vi "Helium Fridge Cool-DownCaitlyn.vi"() -> ()   [LabVIEW 2014]
uses:
  <vilib>/Analysis/8numeric.llb/1D Numeric Integration.vi
  <vilib>/express/express shared/transition.llb/Dynamic To Waveform Array.vi
  <vilib>/express/express signal manip/GetorSetDDTAttributes/Set DDT Attributes/SetT0.vi
  <vilib>/express/express shared/transition.llb/Waveform Array To Dynamic.vi
  <vilib>/express/express signal manip/GetorSetDDTAttributes/Set DDT Attributes/Set DDT Properties.xnode
  <vilib>/Analysis/NI_AALPro.lvlib
panel:
  out "Array - Numeric":dbl[](array[numeric])
  out "Index":dbl
  out "Array Size":dbl
  in  "Boolean":bool
  in  "Wing Fit Subtract":bool=TRUE
  in  "Wing Fit":bool=TRUE
  out "Fit Right X":dbl[](array[numeric])
  out "Fit Left X":dbl[](array[numeric])
  out "Modulator (Y)":dbl[](array[numeric])
  out "Input Triangle (X)":dbl[](array[numeric])
  out "Fit Right Y":dbl[](array[numeric])
  out "Fit Left Y":dbl[](array[numeric])
  out "Fit Right":dbl[](array[numeric])
  out "Fit Left":dbl[](array[numeric])
  in  "Numeric Control":dbl=0.01
  out "NMR.T":dbl
  out "Temp  2":bool
  out "Q Meter Temp":dynamicdata(graph)
  in  "stop 2":bool
  in  "Right wing":dbl
  in  "Left wing":dbl
  in  "Submit":bool
  out "Is Flashing":bool
  in  "Error Beat":bool
  in  "Clear":bool
  in  "Comment":string
  out "Heartbeat":bool
  out "Most Recent Error":string
  out "Baseline Subtracted Integral vs. Time":dbl(graph)
  out "Time of Last Baseline":string
  out "Baseline":dbl[](array[numeric])
  in  "Baseline Subtract":bool
  in  "Get Baseline":bool
  out "Recording":bool
  out "Time of Last Recording":string
  in  "Record \nNMR Sweeps":bool
  in  "Depth/Div\n(kHz)":dbl=10.0
  in  "Central Freq. \n(MHz)":dbl=13.0
  in  "stop (F)":bool caption="Triangle Wave"
  in  "Triangle Wave\nRate (Hz)":dbl=0.3
  out "Time Elapsed \nDuring Sweeps (s)":dbl
  out "Lab Time":string
  out "Most Recent Error (NMR)":string
  out "Last Sweep Start Time":string
  out "Most Recent Error (Temp)":string
  out "Last Measurement Taken":string
  out "VI Start Time":string
  in  "Time Between\nTemp Ponts (s)":dbl=30.0
  out "Temp":bool
  out "NMR":bool
  in  "stop":bool
  out "Input Triangle Wave":dynamicdata(graph)
  out "Modulator":dynamicdata(graph)
  out "NMR":cluster{"Y":dbl[], "Y":dbl[]}[](graph)
  in  "# of Sweeps":dbl=1.0
  out "Resistance Strip Chart":dynamicdata(graph)
  out "Temperature Strip Chart":dynamicdata(graph)
  in  "Heartbeat":bool
  in  "Temp Strip Chart":bool
  out "Errors":bool
  in  "Silence Flashing":bool
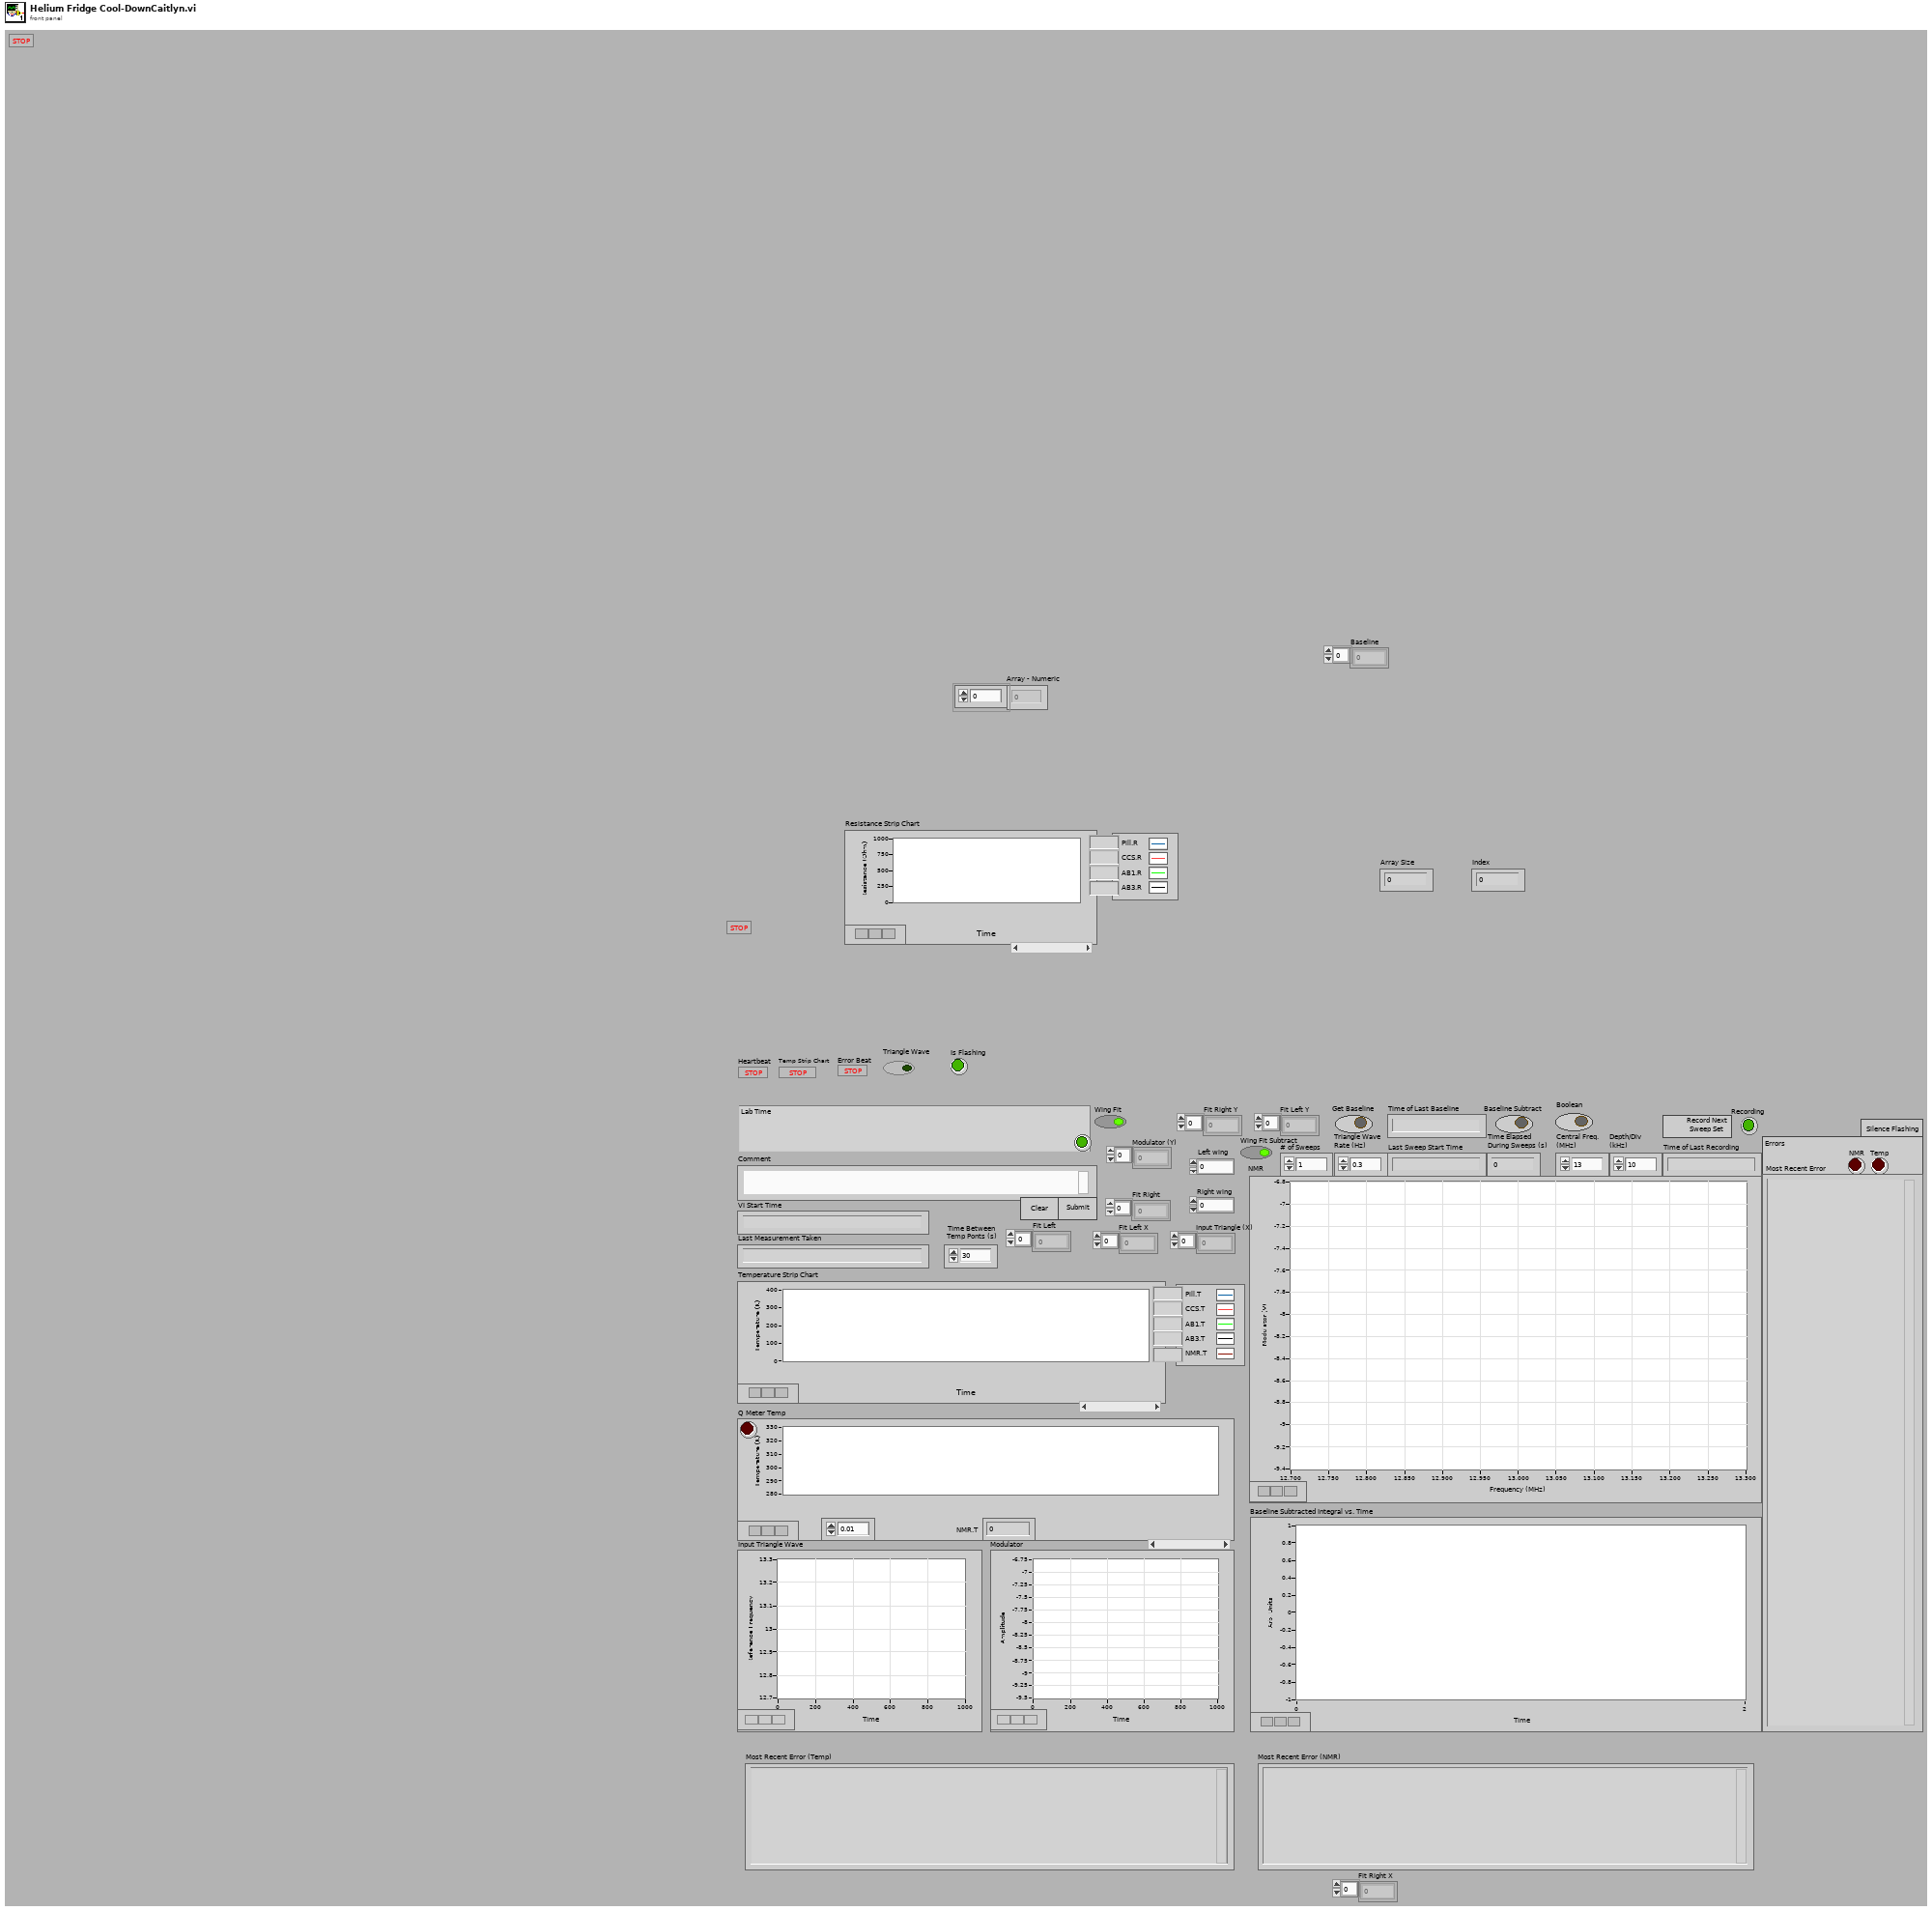
[diagram p1: front panel]
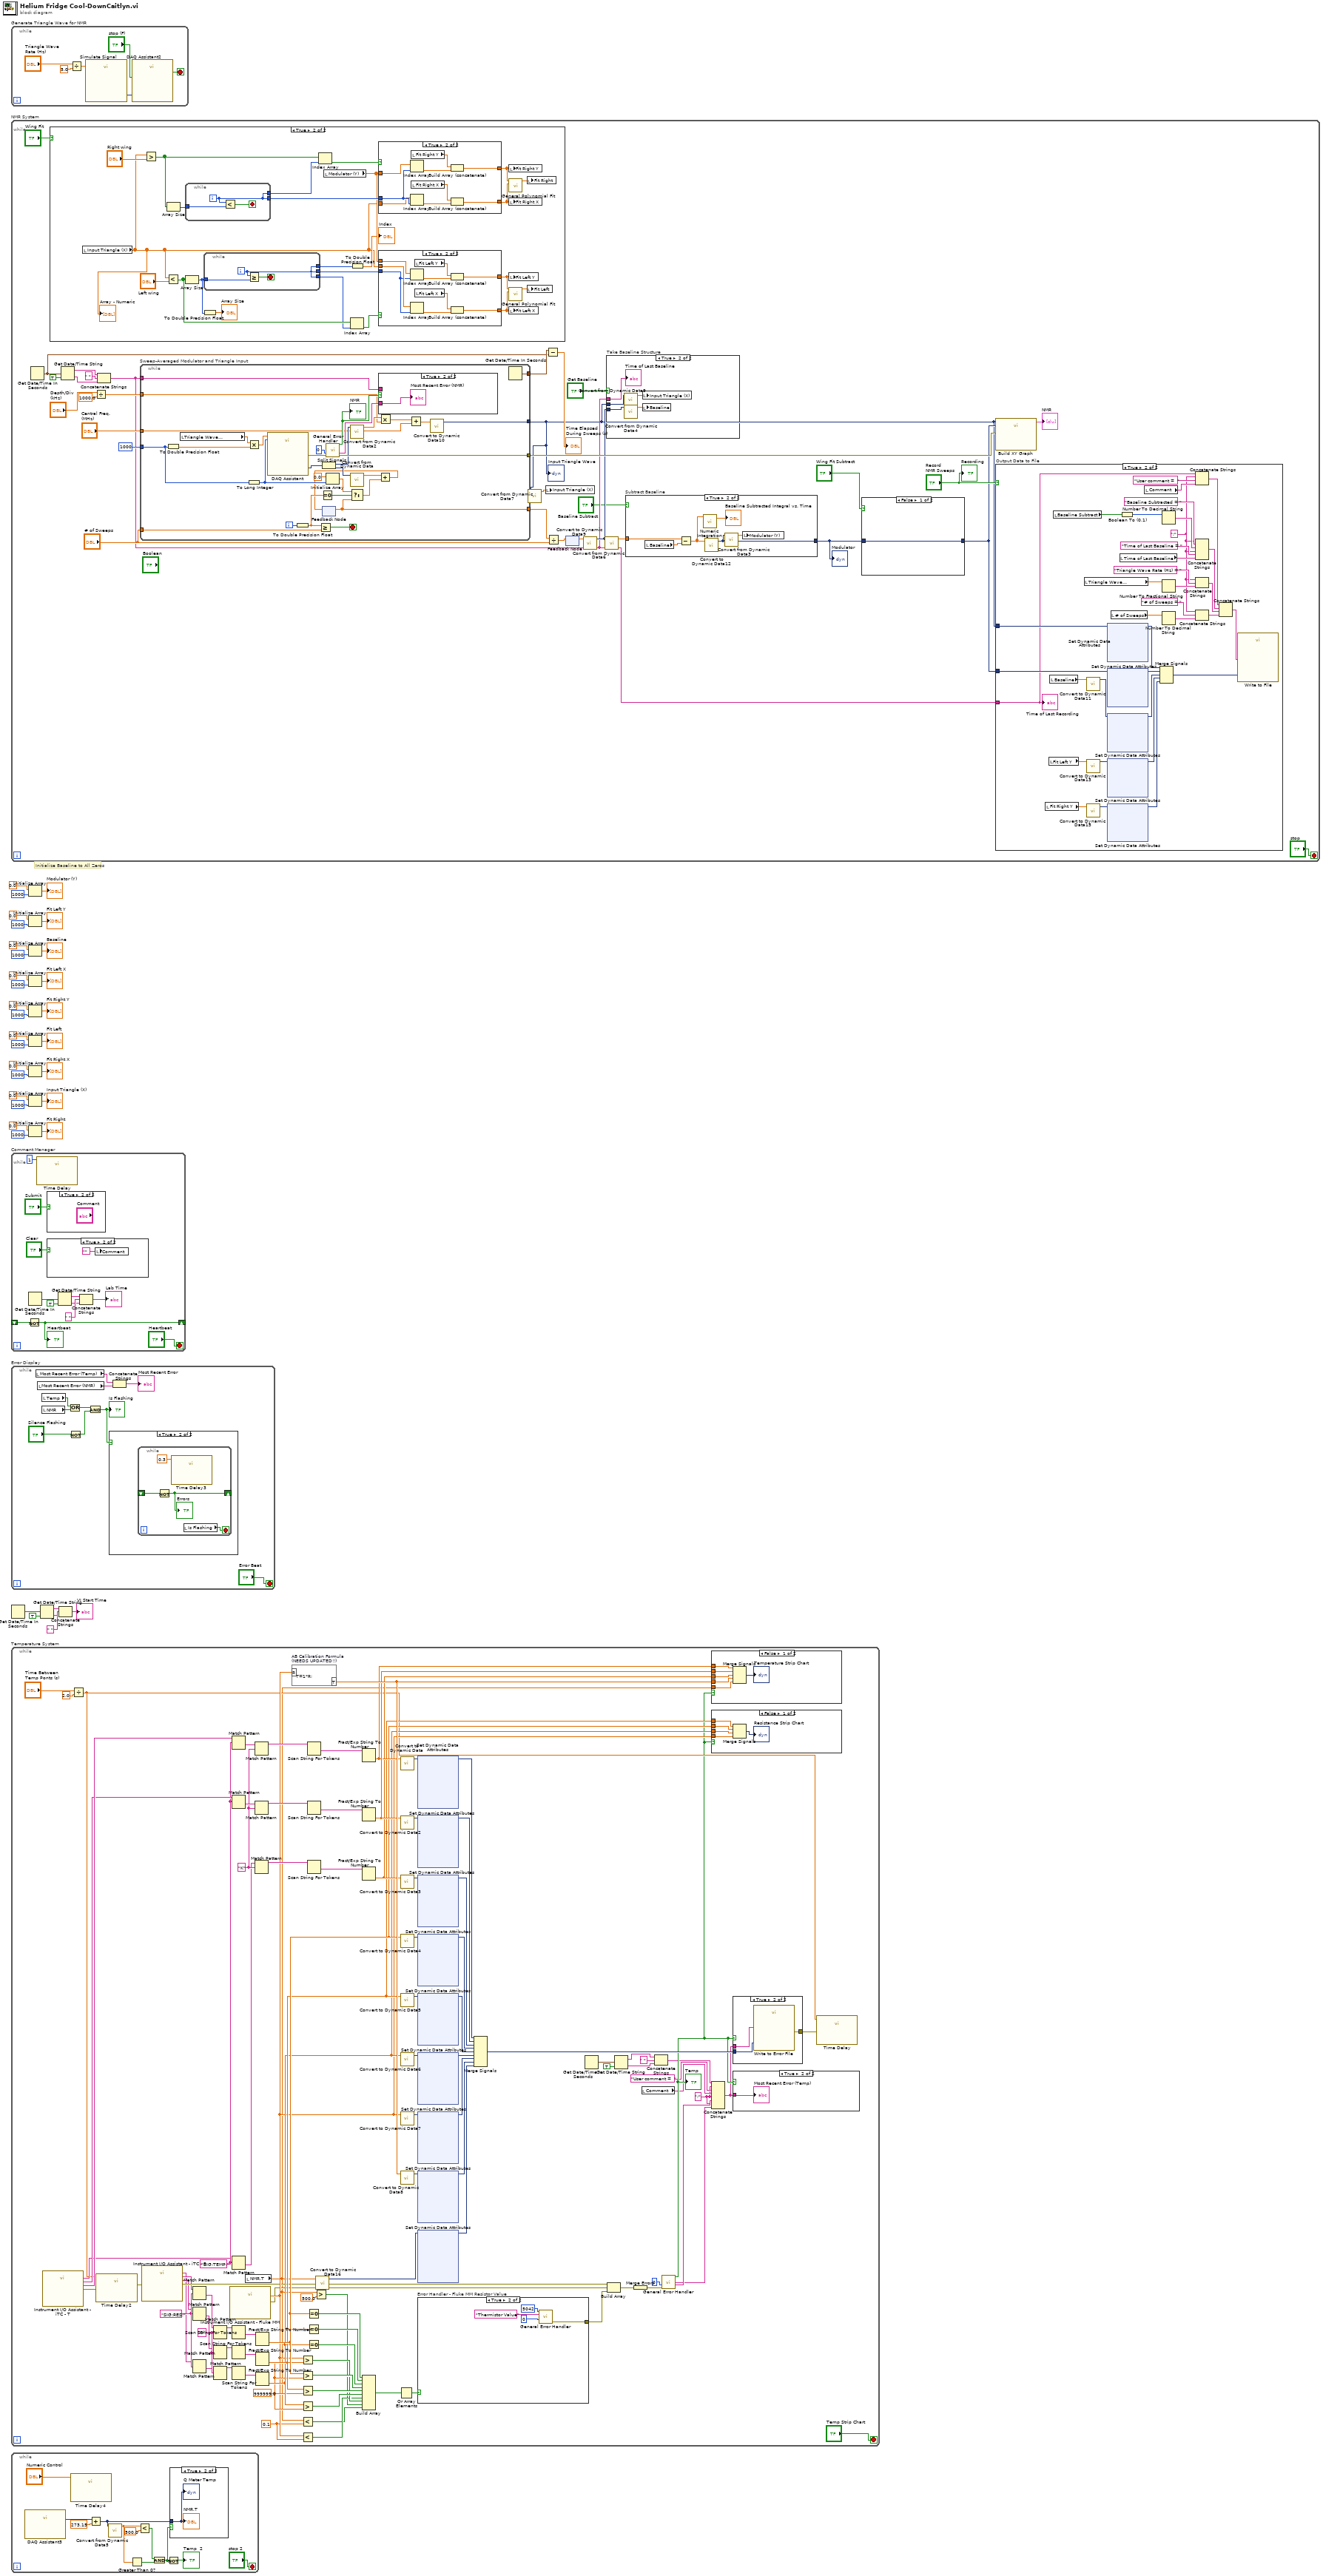
[diagram p0: block diagram]
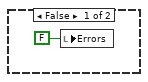
[diagram p3: hidden frame]
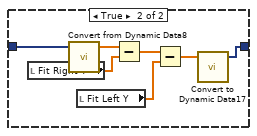
[diagram p4: hidden frame]
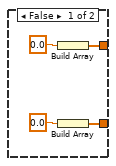
[diagram p6: hidden frame]
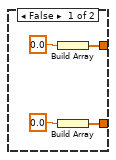
[diagram p7: hidden frame]
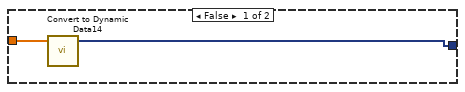
[diagram p8: hidden frame]
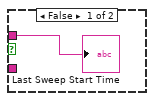
[diagram p11: hidden frame]
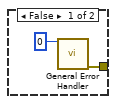
[diagram p14: hidden frame]
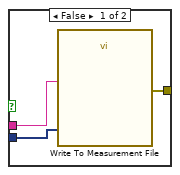
[diagram p17: hidden frame]
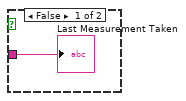
[diagram p18: hidden frame]
diagram:
  # "Initialize Baseline to All Zeros"
  n1 = while "Generate Triangle Wave for NMR" {
    stop <- w38 stop-if-true
    n2 = Divide(x="Triangle Wave\nRate (Hz)", y=5.0) -> (x/y=w34:dbl)
    n3 = call "Simulate Signal"("Frequency"=w34) -> ("Triangle"=w37:dynamicdata)  [unwired: 13 in, 1 out]
    n4 = call "DAQ Assistant2"("data"=w37, "stop (F)"="stop (F)") -> ("stopped"=w38:bool)  [unwired: 15 in, 2 out]
  }
  n5 = while "NMR System" {
    stop <- "stop" stop-if-true
    n6 = Get Date/Time In Seconds() -> (seconds since 1Jan1904=w58:timestamp)
    n7 = case shown="True" "Wing Fit" {
      frame False {
      }
      frame True {
        n8 = local read "Input Triangle (X)"() -> (w79:dbl[])
        "Array - Numeric" <- w79
        n9 = Greater?(x=w79, y="Right wing") -> (0:w97:bool[])
        n10 = Less?(x=w79, y="Left wing") -> (x < y?=w91:bool[])
        n11 = Array Size(array=w97) -> (size(s)=w98:i32)
        n12 = while {
          tunnel: w98 -> [w133]
          tunnel: [w131] -> w99
          tunnel: [w131] -> w101
          i -> [w131]
          stop <- w132 stop-if-true
          n13 = Less?(x=w131, y=w133) -> (x < y?=w132:bool)
        }
        n14 = Array Size(array=w91) -> (size(s)=w84:i32)
        n15 = To Double Precision Float(number=w84) -> (double precision float=→"Array Size":dbl)
        n16 = while {
          tunnel: [w103] -> w82
          tunnel: w84 -> [w104]
          tunnel: [w103] -> w85
          tunnel: [w103] -> w80
          i -> [w103]
          stop <- w102 stop-if-true
          n17 = Greater Or Equal?(x=w103, y=w104) -> (x >= y?=w102:bool)
        }
        n18 = Index Array(array=w97, index=w99) -> (element=w100:bool)
        n19 = local read "Modulator (Y)"() -> (w89:dbl[])
        n20 = Index Array(array=w91, index=w82) -> (element=w90:bool)
        n21 = To Double Precision Float(number=w80) -> (double precision float=→"Index":dbl)
        n22 = case shown="True" w100 {
          tunnel: w101 -> [_ w130]
          tunnel: w79 -> [_ w129]
          tunnel: w89 -> [_ w128]
          tunnel: [w120 w123] -> w95
          tunnel: [w118 w122] -> w93
          frame False {
            n23 = Build Array(0.0) -> (w120:dbl[])
            n24 = Build Array(0.0) -> (w118:dbl[])
          }
          frame True {
            n25 = Index Array(array=w128, index=w130) -> (element=w126:dbl)
            n26 = Index Array(array=w129, index=w130) -> (element=w124:dbl)
            n27 = local read "Fit Right Y"() -> (w127:dbl[])
            n28 = local read "Fit Right X"() -> (w125:dbl[])
            n29 = Build Array (concatenate)(w127, w126) -> (w123:dbl[])
            n30 = Build Array (concatenate)(w125, w124) -> (w122:dbl[])
          }
        }
        n31 = case shown="True" w90 {
          tunnel: w79 -> [_ w117]
          tunnel: w89 -> [_ w116]
          tunnel: w85 -> [_ w115]
          tunnel: [w107 w110] -> w88
          tunnel: [w105 w109] -> w87
          frame False {
            n32 = Build Array(0.0) -> (w107:dbl[])
            n33 = Build Array(0.0) -> (w105:dbl[])
          }
          frame True {
            n34 = Index Array(array=w116, index=w115) -> (element=w112:dbl)
            n35 = Index Array(array=w117, index=w115) -> (element=w113:dbl)
            n36 = local read "Fit Left Y"() -> (w111:dbl[])
            n37 = local read "Fit Left X"() -> (w114:dbl[])
            n38 = Build Array (concatenate)(w111, w112) -> (w110:dbl[])
            n39 = Build Array (concatenate)(w114, w113) -> (w109:dbl[])
          }
        }
        n40 = local write "Fit Right Y"(w95) -> ()
        n41 = call <vilib>:"General Polynomial Fit.vi"("Y"=w95, "X"=w93) -> ("Best Polynomial Fit"=w94:dbl[])  [unwired: 10 in, 3 out]
        n42 = local write "Fit Right X"(w93) -> ()
        n43 = local write "Fit Left Y"(w88) -> ()
        n44 = call <vilib>:"General Polynomial Fit.vi"("Y"=w88, "X"=w87) -> ("Best Polynomial Fit"=w86:dbl[])  [unwired: 10 in, 3 out]
        n45 = local write "Fit Left X"(w87) -> ()
        n46 = local write "Fit Right"(w94) -> ()
        n47 = local write "Fit Left"(w86) -> ()
      }
    }
    n48 = Get Date/Time String(seconds (now)=w58, want seconds? (F)=TRUE) -> (date string=w61:string, time string=w63:string)  [unwired: 1 in]
    n49 = Divide(x="Depth/Div\n(kHz)", y=1000.0) -> (x/y=w52:dbl)
    n50 = Concatenate Strings(w61, " ", w63) -> (w48:string)
    n51 = while "Sweep-Averaged Modulator and Triangle Input" {
      tunnel: "# of Sweeps" -> [w276]
      tunnel: 1000 -> [w275]
      tunnel: [w294] -> w67
      tunnel: w48 -> [w288]
      tunnel: [w287] -> w59
      tunnel: [w285] -> w56
      tunnel: w52 -> [w279]
      tunnel: "Central Freq. \n(MHz)" -> [w278]
      tunnel: [w277] -> w40
      i -> [w300]
      stop <- w293 stop-if-true
      n52 = To Double Precision Float(number=w275) -> (double precision float=w282:dbl)
      n53 = local read "Triangle Wave\nRate (Hz)"() -> (w284:dbl)
      n54 = Multiply(x=w284, y=w282) -> (x*y=w286:dbl)
      n55 = To Long Integer(number=w275) -> (32bit integer=w283:i32)
      n56 = call "DAQ Assistant"("rate"=w286, "number of samples"=w283) -> ("data"=w302:dynamicdata, "error out"=w291:errorcluster)  [unwired: 15 in, 1 out]
      n57 = To Double Precision Float(number=w300) -> (double precision float=w299:dbl)
      n58 = Greater Or Equal?(x=w299, y=w276) -> (x >= y?=w293:bool)
      n59 = Equal To 0?(x=w299) -> (x = 0?=w298:bool)
      n60 = Split Signals(w302) -> (w281:dynamicdata, w301:dynamicdata)  [unwired: 2 in]
      n61 = feedback #1() -> (w294:dbl[])  [unwired: 1 in]
      n62 = call <vilib>:"General Error Handler.vi"("type of dialog (OK msg:1)"=0, "error in (no error)"=w291) -> ("error?"=w289:bool, "message"=w292:string, "error out"=w285:errorcluster)  [unwired: 9 in, 2 out]
      "NMR" <- w289
      n63 = Initialize Array(0.0, w283) -> (w296:dbl[])
      n64 = call "Convert from Dynamic Data2"("Dynamic Data Type"=w281) -> ("Array"=w280:dbl[])  [unwired: 3 in]
      n65 = call "Convert from Dynamic Data"("Dynamic Data Type"=w301) -> ("Array"=w295:dbl[])  [unwired: 3 in]
      n66 = Select(t=w296, s=w298, f=w294) -> (s? t:f=w297:dbl[])
      n67 = case shown="True" w289 {
        tunnel: w292 -> [_ w305]
        tunnel: w288 -> [w304 _]
        frame False {
          "Last Sweep Start Time" <- w304
        }
        frame True {
          "Most Recent Error (NMR)" <- w305
        }
      }
      n68 = Add(x=w295, y=w297) -> (x+y=w272:dbl[])
      n69 = feedback-in #1(w272) -> ()
      n70 = Multiply(x=w280, y=w279) -> (x*y=w273:dbl[])
      n71 = Add(x=w273, y=w278) -> (x+y=w274:dbl[])
      n72 = call "Convert to Dynamic Data10"("Array"=w274) -> ("Dynamic Data Type"=w277:dynamicdata)  [unwired: 3 in]
      n73 = Get Date/Time In Seconds() -> (seconds since 1Jan1904=w287:timestamp)
    }
    "Input Triangle Wave" <- w40
    n74 = call "Convert from Dynamic Data7"("Dynamic Data Type"=w40) -> ("Array"=w41:dbl[])  [unwired: 3 in]
    n75 = local write "Input Triangle (X)"(w41) -> ()
    n76 = Subtract(x=w59, y=w58) -> (x-y=→"Time Elapsed \nDuring Sweeps (s)":dbl)
    n77 = Divide(x=w67, y="# of Sweeps") -> (x/y=w65:dbl[])
    n78 = feedback-in #2(w65) -> ()
    n79 = feedback #2() -> (w64:dbl[])  [unwired: 1 in]
    n80 = call "Convert to Dynamic Data9"("Array"=w64) -> ("Dynamic Data Type"=w49:dynamicdata)  [unwired: 3 in]
    n81 = call "Convert from Dynamic Data6"("Dynamic Data Type"=w49) -> ("Array"=w46:dbl[])  [unwired: 3 in]
    n82 = case "Take Baseline Structure" shown="True" "Get Baseline" {
      tunnel: w49 -> [_ w146]
      tunnel: w48 -> [_ w144]
      tunnel: w40 -> [_ w143]
      frame False {
      }
      frame True {
        n83 = call "Convert from Dynamic Data9"("Dynamic Data Type"=w143) -> ("Array"=w142:dbl[])  [unwired: 3 in]
        n84 = call "Convert from Dynamic Data4"("Dynamic Data Type"=w146) -> ("Array"=w145:dbl[])  [unwired: 3 in]
        n85 = local write "Input Triangle (X)"(w142) -> ()
        n86 = local write "Baseline"(w145) -> ()
        "Time of Last Baseline" <- w144
      }
    }
    n87 = case "Subtract Baseline" shown="True" "Baseline Subtract" {
      tunnel: w46 -> [w135 w140]
      tunnel: [w134 w137] -> w44
      frame False {
        n88 = call "Convert to Dynamic Data14"("Array"=w135) -> ("Dynamic Data Type"=w134:dynamicdata)  [unwired: 3 in]
      }
      frame True {
        n89 = local read "Baseline"() -> (w141:dbl[])
        n90 = Subtract(x=w140, y=w141) -> (x-y=w138:dbl[])
        n91 = call-poly <vilib>:"Numeric Integration.vi"("Input Array"=w138) -> ("result"=→"Baseline Subtracted Integral vs. Time":dbl)  [unwired: 2 in, 1 out]
        n92 = call "Convert to Dynamic Data12"("Array"=w138) -> ("Dynamic Data Type"=w137:dynamicdata)  [unwired: 3 in]
        n93 = call "Convert from Dynamic Data3"("Dynamic Data Type"=w137) -> ("Array"=w136:dbl[])  [unwired: 3 in]
        n94 = local write "Modulator (Y)"(w136) -> ()
      }
    }
    "Modulator" <- w44
    n95 = case shown="False" "Wing Fit Subtract" {
      tunnel: w44 -> [w71 w78]
      tunnel: [w71 w72] -> w43
      frame False {
      }
      frame True {
        n96 = local read "Fit Right Y"() -> (w76:dbl[])
        n97 = call "Convert from Dynamic Data8"("Dynamic Data Type"=w78) -> ("Array"=w77:dbl[])  [unwired: 3 in]
        n98 = local read "Fit Left Y"() -> (w74:dbl[])
        n99 = Subtract(x=w77, y=w76) -> (x-y=w75:dbl[])
        n100 = Subtract(x=w75, y=w74) -> (x-y=w73:dbl[])
        n101 = call "Convert to Dynamic Data17"("Array"=w73) -> ("Dynamic Data Type"=w72:dynamicdata)  [unwired: 3 in]
      }
    }
    n102 = call "Build XY Graph"("error in (no error)"=w56, "Y Input"=w43, "X Input"=w40) -> ("XY Graph"=→"NMR":cluster{"Y":dbl[], "Y":dbl[]}[])  [unwired: 7 in, 1 out]
    n103 = case "Output Data to File" shown="True" "Record \nNMR Sweeps" {
      tunnel: w48 -> [_ w170]
      tunnel: w43 -> [_ w177]
      tunnel: w40 -> [_ w176]
      frame False {
      }
      frame True {
        w154 = ";"
        n104 = local read "Fit Right Y"() -> (w149:dbl[])
        n105 = local read "Fit Left Y"() -> (w151:dbl[])
        n106 = local read "Baseline"() -> (w175:dbl[])
        n107 = local read "Baseline Subtract"() -> (w172:bool)
        n108 = local read "Triangle Wave\nRate (Hz)"() -> (w173:dbl)
        n109 = call "Convert to Dynamic Data11"("Array"=w175) -> ("Dynamic Data Type"=w174:dynamicdata)  [unwired: 3 in]
        n110 = call "Convert to Dynamic Data13"("Array"=w151) -> ("Dynamic Data Type"=w150:dynamicdata)  [unwired: 3 in]
        n111 = call "Convert to Dynamic Data15"("Array"=w149) -> ("Dynamic Data Type"=w148:dynamicdata)  [unwired: 3 in]
        n112 = xnode "Set Dynamic Data Attributes"("Signals In"=w176) -> ("Signals Out"=w181:dynamicdata)  [unwired: 4 in, 1 out]
        n113 = xnode "Set Dynamic Data Attributes"("Signals In"=w177) -> ("Signals Out"=w179:dynamicdata)  [unwired: 4 in, 1 out]
        n114 = xnode "Set Dynamic Data Attributes"("Signals In"=w174) -> ("Signals Out"=w153:dynamicdata)  [unwired: 4 in, 1 out]
        n115 = xnode "Set Dynamic Data Attributes"("Signals In"=w150) -> ("Signals Out"=w152:dynamicdata)  [unwired: 4 in, 1 out]
        n116 = xnode "Set Dynamic Data Attributes"("Signals In"=w148) -> ("Signals Out"=w147:dynamicdata)  [unwired: 4 in, 1 out]
        n117 = local read "# of Sweeps"() -> (w178:dbl)
        n118 = local read "Time of Last Baseline"() -> (w159:string)
        n119 = Boolean To (0,1)(Boolean=w172) -> (0, 1=w171:i16)
        n120 = local read "Comment"() -> (w168:string)
        n121 = Merge Signals(w181, w179, w153, w152, w147) -> (w180:dynamicdata)
        n122 = Number To Decimal String(number=w171) -> (decimal integer string=w164:string)  [unwired: 1 in]
        n123 = Number To Fractional String(number=w173) -> (F-format string=w162:string)  [unwired: 3 in]
        n124 = Number To Decimal String(number=w178) -> (decimal integer string=w166:string)  [unwired: 1 in]
        n125 = Concatenate Strings(w170, w154, "User comment =  ", w168) -> (w161:string)
        n126 = Concatenate Strings(w154, "Baseline Subtracted = ", w164, w154, "Time of Last Baseline = ", w159) -> (w158:string)
        n127 = Concatenate Strings(w154, "Triangle Wave Rate (Hz) = ", w162) -> (w157:string)
        n128 = Concatenate Strings(w154, "# of Sweeps = ", w166) -> (w156:string)
        n129 = Concatenate Strings(w161, w158, w157, w156) -> (w155:string)
        n130 = call "Write to File"("Signals"=w180, "Comment"=w155) -> ()  [unwired: 15 in, 3 out]
        "Time of Last Recording" <- w170
      }
    }
    "Recording" <- "Record \nNMR Sweeps"
  }
  n131 = while "Comment Manager" {
    shift-right: [w314] -> _
    shift-left: _ -> [w317]
    stop <- "Heartbeat" stop-if-true
    n132 = Not(x=w317) -> (.not. x?=w314:bool)
    "Heartbeat" <- w314
    n133 = Get Date/Time In Seconds() -> (seconds since 1Jan1904=w312:timestamp)
    n134 = call "Time Delay"("Delay Time (s)"=1) -> ()  [unwired: 10 in, 1 out]
    n135 = case shown="True" "Submit" {
      frame False {
      }
      frame True {
      }
    }
    n136 = case shown="True" "Clear" {
      frame False {
      }
      frame True {
        n137 = local write "Comment"("") -> ()
      }
    }
    n138 = Get Date/Time String(seconds (now)=w312, want seconds? (F)=TRUE) -> (date string=w311:string, time string=w309:string)  [unwired: 1 in]
    n139 = Concatenate Strings(w311, " ", w309) -> (→"Lab Time":string)
  }
  n140 = while "Error Display" {
    stop <- "Error Beat" stop-if-true
    n141 = local read "Most Recent Error (Temp)"() -> (w319:string)
    n142 = local read "Most Recent Error (NMR)"() -> (w320:string)
    n143 = local read "Temp"() -> (w328:bool)
    n144 = local read "NMR"() -> (w327:bool)
    n145 = Or(x=w328, y=w327) -> (x .or. y?=w325:bool)
    n146 = Not(x="Silence Flashing") -> (.not. x?=w323:bool)
    n147 = And(x=w325, y=w323) -> (x .and. y?=w322:bool)
    "Is Flashing" <- w322
    n148 = case shown="True" w322 {
      frame False {
        n149 = local write "Errors"(FALSE) -> ()
      }
      frame True {
        n150 = while {
          shift-right: [w331] -> _
          shift-left: _ -> [w333]
          stop <- w330 stop-if-true
          n151 = Not(x=w333) -> (.not. x?=w331:bool)
          "Errors" <- w331
          n152 = call "Time Delay3"("Delay Time (s)"=0.3) -> ()  [unwired: 10 in, 1 out]
          n153 = local read "Is Flashing"() -> (w330:bool)
        }
      }
    }
    n154 = Concatenate Strings(w319, w320) -> (→"Most Recent Error":string)
  }
  n155 = Get Date/Time In Seconds() -> (seconds since 1Jan1904=w32:timestamp)
  n156 = while "Temperature System" {
    stop <- "Temp Strip Chart" stop-if-true
    w341 = ";"
    w336 = 0.1
    w364 = 999999.0
    w400 = "O"
    w401 = "SIG:RES:"
    w407 = "SIG:TEMP:"
    w406 = "K"
    n157 = call "Instrument I/O Assistant - iTC - T"() -> ("AB1.T"=w405:string, "CCS.T"=w410:string, "Pill.T"=w413:string, "error out"=w355:errorcluster)  [unwired: 23 in, 1 out]
    n158 = Divide(x="Time Between\nTemp Ponts (s)", y=2.0) -> (x/y=w350:dbl)
    n159 = call "Time Delay2"("error in (no error)"=w355, "Delay Time (s)"=w350) -> ("error out"=w356:errorcluster)  [unwired: 9 in]
    n160 = call "Instrument I/O Assistant - iTC - R"("error in"=w356) -> ("AB1.R"=w352:string, "CCS.R"=w353:string, "Pill.R"=w354:string, "error out"=w357:errorcluster)  [unwired: 22 in, 1 out]
    n161 = Match Pattern(string=w353, regular expression=w401) -> (after substring=w399:string)  [unwired: 1 in, 3 out]
    n162 = Match Pattern(string=w354, regular expression=w401) -> (after substring=w398:string)  [unwired: 1 in, 3 out]
    n163 = Match Pattern(string=w352, regular expression=w401) -> (after substring=w397:string)  [unwired: 1 in, 3 out]
    n164 = Match Pattern(string=w399, regular expression=w400) -> (before substring=w396:string)  [unwired: 1 in, 3 out]
    n165 = Match Pattern(string=w398, regular expression=w400) -> (before substring=w395:string)  [unwired: 1 in, 3 out]
    n166 = Match Pattern(string=w397, regular expression=w400) -> (before substring=w394:string)  [unwired: 1 in, 3 out]
    n167 = call "Instrument I/O Assistant - Fluke MM"() -> ("AB3.R"=w362:dbl, "error out"=w360:errorcluster)  [unwired: 25 in, 1 out]
    n168 = Match Pattern(string=w413, regular expression=w407) -> (after substring=w412:string)  [unwired: 1 in, 3 out]
    n169 = Match Pattern(string=w410, regular expression=w407) -> (after substring=w409:string)  [unwired: 1 in, 3 out]
    n170 = Match Pattern(string=w405, regular expression=w407) -> (after substring=w404:string)  [unwired: 1 in, 3 out]
    n171 = Scan String For Tokens(9:w396) -> (1:w393:string)  [unwired: 5 in, 3 out]
    n172 = Scan String For Tokens(9:w395) -> (1:w392:string)  [unwired: 5 in, 3 out]
    n173 = Scan String For Tokens(9:w394) -> (1:w391:string)  [unwired: 5 in, 3 out]
    n174 = local read "NMR.T"() -> (w334:dbl)
    n175 = Match Pattern(string=w412, regular expression=w406) -> (before substring=w411:string)  [unwired: 1 in, 3 out]
    n176 = Match Pattern(string=w409, regular expression=w406) -> (before substring=w408:string)  [unwired: 1 in, 3 out]
    n177 = Match Pattern(string=w404, regular expression=w406) -> (before substring=w403:string)  [unwired: 1 in, 3 out]
    n178 = Fract/Exp String To Number(string=w393) -> (number=w370:dbl)  [unwired: 3 in, 1 out]
    n179 = Fract/Exp String To Number(string=w392) -> (number=w369:dbl)  [unwired: 3 in, 1 out]
    n180 = Fract/Exp String To Number(string=w391) -> (number=w368:dbl)  [unwired: 3 in, 1 out]
    n181 = formula code="T=1*R;" "AB Calibration Formula\n(NEEDS UPDATED!!)"("R"=w362) -> ("T"=w381:dbl)
    n182 = Greater?(x=w362, y=w364) -> (0:w363:bool)
    n183 = Greater?(x=w370, y=w364) -> (0:w367:bool)
    n184 = Greater?(x=w369, y=w364) -> (0:w366:bool)
    n185 = Greater?(x=w368, y=w364) -> (0:w365:bool)
    n186 = Less?(x=w334, y=w336) -> (x < y?=w335:bool)
    n187 = Less?(x=w362, y=w336) -> (x < y?=w361:bool)
    n188 = Scan String For Tokens(9:w411) -> (1:w430:string)  [unwired: 5 in, 3 out]
    n189 = Scan String For Tokens(9:w408) -> (1:w428:string)  [unwired: 5 in, 3 out]
    n190 = Scan String For Tokens(9:w403) -> (1:w427:string)  [unwired: 5 in, 3 out]
    n191 = Equal To 0?(x=w370) -> (x = 0?=w378:bool)
    n192 = Equal To 0?(x=w369) -> (x = 0?=w377:bool)
    n193 = Equal To 0?(x=w368) -> (x = 0?=w376:bool)
    n194 = Greater?(x=w334, y=500.0) -> (0:w337:bool)
    n195 = call "Convert to Dynamic Data16"("Double"=w334) -> ("Dynamic Data Type"=w340:dynamicdata)  [unwired: 3 in]
    n196 = Fract/Exp String To Number(string=w430) -> (number=w372:dbl)  [unwired: 3 in, 1 out]
    n197 = Fract/Exp String To Number(string=w428) -> (number=w373:dbl)  [unwired: 3 in, 1 out]
    n198 = Fract/Exp String To Number(string=w427) -> (number=w371:dbl)  [unwired: 3 in, 1 out]
    n199 = Build Array(w378, w377, w376, w367, w366, w365, w361, w363, w337, w335) -> (w375:bool[])
    n200 = Or Array Elements(Boolean array=w375) -> (logical OR=w374:bool)
    n201 = call "Convert to Dynamic Data"("Double"=w372) -> ("Dynamic Data Type"=w421:dynamicdata)  [unwired: 3 in]
    n202 = call "Convert to Dynamic Data2"("Double"=w373) -> ("Dynamic Data Type"=w419:dynamicdata)  [unwired: 3 in]
    n203 = call "Convert to Dynamic Data3"("Double"=w371) -> ("Dynamic Data Type"=w418:dynamicdata)  [unwired: 3 in]
    n204 = call "Convert to Dynamic Data4"("Double"=w370) -> ("Dynamic Data Type"=w390:dynamicdata)  [unwired: 3 in]
    n205 = call "Convert to Dynamic Data5"("Double"=w369) -> ("Dynamic Data Type"=w389:dynamicdata)  [unwired: 3 in]
    n206 = call "Convert to Dynamic Data6"("Double"=w368) -> ("Dynamic Data Type"=w388:dynamicdata)  [unwired: 3 in]
    n207 = call "Convert to Dynamic Data7"("Double"=w362) -> ("Dynamic Data Type"=w384:dynamicdata)  [unwired: 3 in]
    n208 = call "Convert to Dynamic Data8"("Double"=w381) -> ("Dynamic Data Type"=w380:dynamicdata)  [unwired: 3 in]
    n209 = xnode "Set Dynamic Data Attributes"("Signals In"=w421) -> ("Signals Out"=w420:dynamicdata)  [unwired: 4 in, 1 out]
    n210 = xnode "Set Dynamic Data Attributes"("Signals In"=w419) -> ("Signals Out"=w417:dynamicdata)  [unwired: 4 in, 1 out]
    n211 = xnode "Set Dynamic Data Attributes"("Signals In"=w418) -> ("Signals Out"=w416:dynamicdata)  [unwired: 4 in, 1 out]
    n212 = xnode "Set Dynamic Data Attributes"("Signals In"=w390) -> ("Signals Out"=w387:dynamicdata)  [unwired: 4 in, 1 out]
    n213 = xnode "Set Dynamic Data Attributes"("Signals In"=w389) -> ("Signals Out"=w386:dynamicdata)  [unwired: 4 in, 1 out]
    n214 = xnode "Set Dynamic Data Attributes"("Signals In"=w388) -> ("Signals Out"=w385:dynamicdata)  [unwired: 4 in, 1 out]
    n215 = xnode "Set Dynamic Data Attributes"("Signals In"=w384) -> ("Signals Out"=w383:dynamicdata)  [unwired: 4 in, 1 out]
    n216 = xnode "Set Dynamic Data Attributes"("Signals In"=w380) -> ("Signals Out"=w379:dynamicdata)  [unwired: 4 in, 1 out]
    n217 = xnode "Set Dynamic Data Attributes"("Signals In"=w340) -> ("Signals Out"=w339:dynamicdata)  [unwired: 4 in, 1 out]
    n218 = case "Error Handler - Fluke MM Resistor Value" shown="True" w374 {
      tunnel: [w449 w454] -> w359
      frame False {
        n219 = call <vilib>:"General Error Handler.vi"("[error code] (0)"=0) -> ("error out"=w449:errorcluster)  [unwired: 10 in, 4 out]
      }
      frame True {
        n220 = call <vilib>:"General Error Handler.vi"("[error code] (0)"=5042, "[error source] (\" \")"="Thermistor Value", "type of dialog (OK msg:1)"=0) -> ("error out"=w454:errorcluster)  [unwired: 8 in, 4 out]
      }
    }
    n221 = Merge Signals(w420, w417, w416, w387, w386, w385, w383, w379, w339) -> (w415:dynamicdata)
    n222 = Get Date/Time In Seconds() -> (seconds since 1Jan1904=w426:timestamp)
    n223 = Build Array(w357, w360, w359) -> (w358:errorcluster[])
    n224 = Get Date/Time String(seconds (now)=w426, want seconds? (F)=TRUE) -> (date string=w424:string, time string=w422:string)  [unwired: 1 in]
    n225 = Merge Errors(w358) -> (w382:errorcluster)
    n226 = local read "Comment"() -> (w346:string)
    n227 = Concatenate Strings(w424, " ", w422) -> (w342:string)
    n228 = call <vilib>:"General Error Handler.vi"("type of dialog (OK msg:1)"=0, "error in (no error)"=w382) -> ("error?"=w349:bool, "source out"=w343:string, "message"=w345:string)  [unwired: 9 in, 2 out]
    "Temp" <- w349
    n229 = case shown="False" w349 {
      tunnel: w372 -> [w555 _]
      tunnel: w373 -> [w554 _]
      tunnel: w371 -> [w553 _]
      tunnel: w381 -> [w552 _]
      tunnel: w334 -> [w550 _]
      frame False {
        n230 = Merge Signals(w555, w554, w553, w552, w550) -> (→"Temperature Strip Chart":dynamicdata)
      }
      frame True {
      }
    }
    n231 = case shown="False" w349 {
      tunnel: w369 -> [w549 _]
      tunnel: w370 -> [w548 _]
      tunnel: w368 -> [w547 _]
      tunnel: w362 -> [w546 _]
      frame False {
        n232 = Merge Signals(w549, w548, w547, w546) -> (→"Resistance Strip Chart":dynamicdata)
      }
      frame True {
      }
    }
    n233 = Concatenate Strings(w342, w341, "User comment =  ", w346, w341, w345, w341, w343) -> (w344:string)
    n234 = case shown="True" w349 {
      tunnel: w415 -> [w558 w561]
      tunnel: w344 -> [w557 w560]
      tunnel: [w556 w559] -> w402
      frame False {
        n235 = call "Write To Measurement File"("Signals"=w558, "Comment"=w557) -> ("error out"=w556:errorcluster)  [unwired: 15 in, 2 out]
      }
      frame True {
        n236 = call "Write to Error File"("Signals"=w561, "Comment"=w560) -> ("error out"=w559:errorcluster)  [unwired: 15 in, 2 out]
      }
    }
    n237 = case shown="True" w349 {
      tunnel: w344 -> [w616 w617]
      frame False {
        "Last Measurement Taken" <- w616
      }
      frame True {
        "Most Recent Error (Temp)" <- w617
      }
    }
    n238 = call "Time Delay"("error in (no error)"=w402, "Delay Time (s)"=w350) -> ()  [unwired: 9 in, 1 out]
  }
  n239 = while {
    stop <- "stop 2" stop-if-true
    n240 = call "DAQ Assistant3"() -> ("data"=w622:dynamicdata)  [unwired: 17 in, 2 out]
    n241 = call "Time Delay4"("Delay Time (s)"="Numeric Control") -> ()  [unwired: 10 in, 1 out]
    n242 = Add(x=w622, y=273.15) -> (x+y=w620:dynamicdata)
    n243 = call "Convert from Dynamic Data5"("Dynamic Data Type"=w620) -> ("Scalar"=w618:dbl)  [unwired: 3 in]
    n244 = Greater Than 0?(x=w618) -> (x > 0?=w619:bool)
    n245 = Less?(x=w618, y=500.0) -> (x < y?=w626:bool)
    n246 = And(x=w626, y=w619) -> (x .and. y?=w624:bool)
    n247 = Not(x=w624) -> (.not. x?=→"Temp  2":bool)
    n248 = case shown="True" w624 {
      tunnel: w620 -> [_ w629]
      frame False {
      }
      frame True {
        "Q Meter Temp" <- w629
        "NMR.T" <- w629
      }
    }
  }
  n249 = Initialize Array(0.0, 1000) -> (→"Modulator (Y)":dbl[])
  n250 = Initialize Array(0.0, 1000) -> (→"Fit Left Y":dbl[])
  n251 = Initialize Array(0.0, 1000) -> (→"Baseline":dbl[])
  n252 = Initialize Array(0.0, 1000) -> (→"Fit Left X":dbl[])
  n253 = Initialize Array(0.0, 1000) -> (→"Fit Right Y":dbl[])
  n254 = Initialize Array(0.0, 1000) -> (→"Fit Left":dbl[])
  n255 = Initialize Array(0.0, 1000) -> (→"Fit Right X":dbl[])
  n256 = Initialize Array(0.0, 1000) -> (→"Input Triangle (X)":dbl[])
  n257 = Initialize Array(0.0, 1000) -> (→"Fit Right":dbl[])
  n258 = Get Date/Time String(seconds (now)=w32, want seconds? (F)=TRUE) -> (date string=w31:string, time string=w29:string)  [unwired: 1 in]
  n259 = Concatenate Strings(w31, " ", w29) -> (→"VI Start Time":string)
